vi "Initialize Front Panel.vi"(8 "error in (no error)":errorcluster, 11 "Test Executive Builder View in":refnum<class "Test Executive Builder View.lvclass">) -> (0 "error out":errorcluster, 3 "Test Executive Builder View out":refnum<class "Test Executive Builder View.lvclass">)   [LabVIEW 2017, in "Test Executive Builder View.lvclass"]
doc: "<License>\nCopyright © 2017 Composed Systems, LLC | All rights reserved\nwww.composed.io\n\nAuthor: Ethan Stern <ethan.stern@composed.io>\n\nThis software is provided \"AS IS\" WITHOUT WARRANTIES, either express or implied, AND IS FOR EDUCATIONAL PURPOSES ONLY.\n</License>"
uses:
  Test Executive Builder View.lvclass
  <vilib>/gpm_packages/@cs/mva-viewable/Source/IViewable/IViewable/IViewable.lvclass
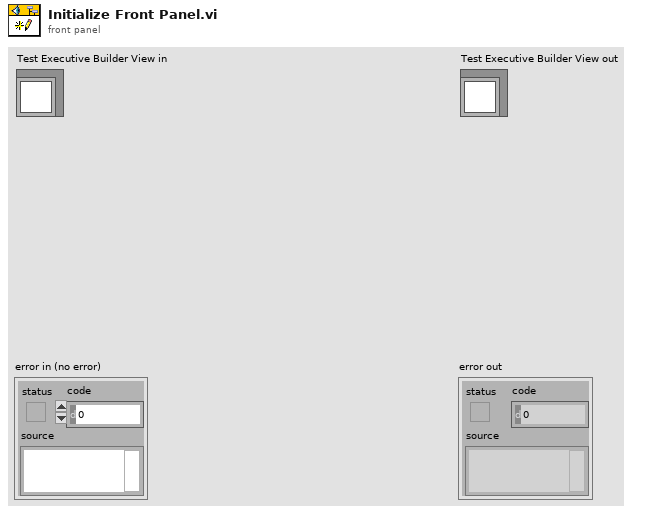
[diagram p1: front panel]
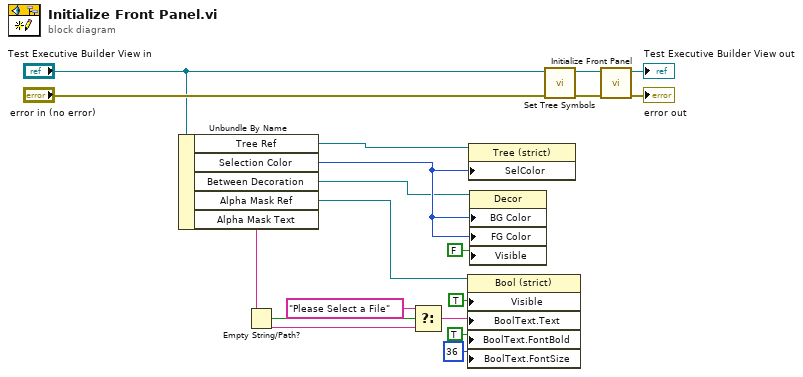
[diagram p0: block diagram]
diagram:
  n1 = Unbundle By Name("Test Executive Builder View in") -> ("Tree Ref"=w12:refnum<vi>, "Selection Color"=w11:u32, "Between Decoration"=w10:refnum<vi>, "Alpha Mask Ref"=w8:refnum<vi>, "Alpha Mask Text"=w5:string)
  n2 = Empty String/Path?(string/path=w5) -> (empty?=w6:bool)
  n3 = Select(t="Please Select a File", s=w6, f=w5) -> (s? t:f=w3:string)
  n4 = property class="Bool (strict)"(reference=w8, "Visible"=TRUE, "BoolText.Text"=w3, "BoolText.FontBold"=TRUE ("Boolean Text.Font:Bold"), "BoolText.FontSize"=u32 36 ("Boolean Text.Font:Size")) -> ()  [unwired: 1 in, 2 out]
  n5 = property class="Tree (strict)"(reference=w12, "SelColor"=w11) -> ()  [unwired: 1 in, 2 out]
  n6 = property class="Decor"(reference=w10, "BG Color"=w11, "FG Color"=w11, "Visible"=FALSE) -> ()  [unwired: 1 in, 2 out]
  n7 = call-dynamic "Set Tree Symbols.vi"("error in (no error)"="error in (no error)", "Test Executive Builder View in"="Test Executive Builder View in") -> ("error out"=w14:errorcluster, "Test Executive Builder View out"=w16:refnum<class "Test Executive Builder View.lvclass">)  [unwired: 8 in]
  n8 = call-parent "Initialize Front Panel.vi"("error in (no error)"=w14, "IViewable in"=w16) -> ("error out"=→"error out":errorcluster, "IViewable out"=→"Test Executive Builder View out":refnum<class "Test Executive Builder View.lvclass">)  [unwired: 8 in]
